vi "LVJSON Pop.vi"(8 "error in (no error)":errorcluster, 10 "Root Path ([]=Root)":string[](array[string]), 11 "Root Element in":T1) -> (0 "error out":errorcluster, 1 "Element out":T1, 2 "Exists?":bool, 3 "Root Element out":T1)   [LabVIEW 2018, in "labview_json.lvlib"]
uses:
  labview_json.lvlib
  Element Type.ctl
  Element.ctl
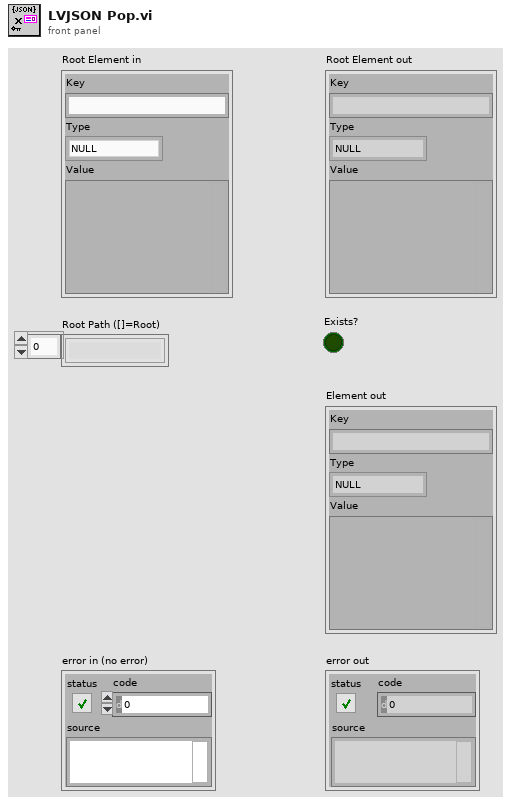
[diagram p1: front panel]
types:
  T1 = typedef "labview_json.lvlib/Element.ctl" = cluster{"Key":string, "Type":T2, "Value":variant}
  T2 = typedef "labview_json.lvlib/Element Type.ctl" = enum8{"NULL", "BOOL", "INT", "UINT", "FLOAT", "STRING", "ARRAY", "OBJECT", "SKIP"}
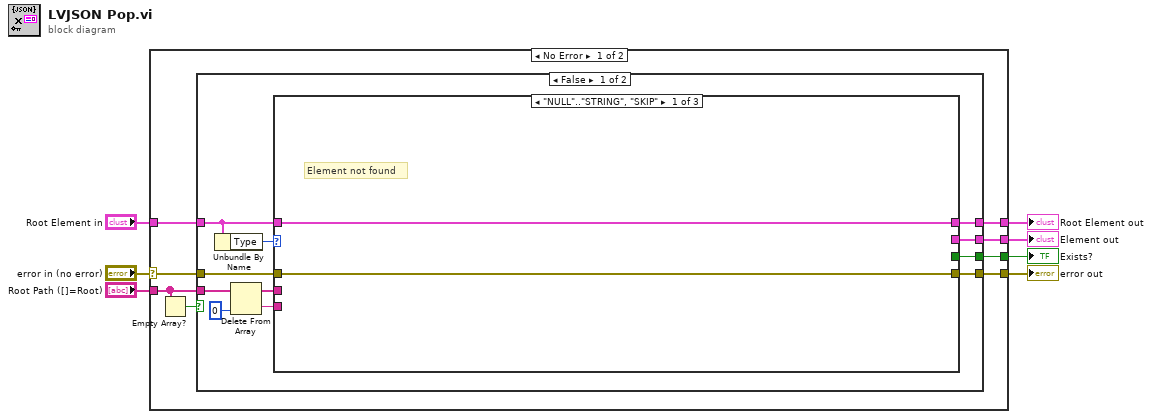
[diagram p0: block diagram]
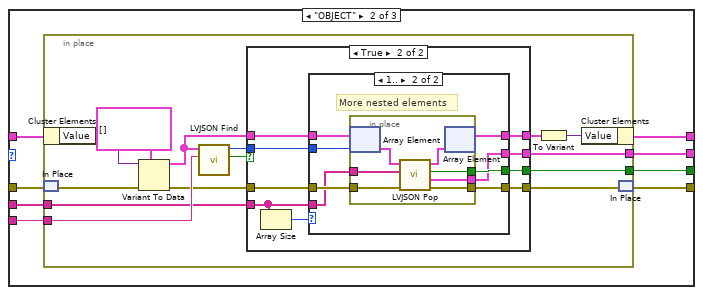
[diagram p2: hidden frame]
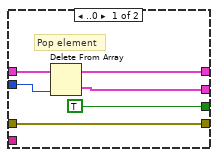
[diagram p4: hidden frame]
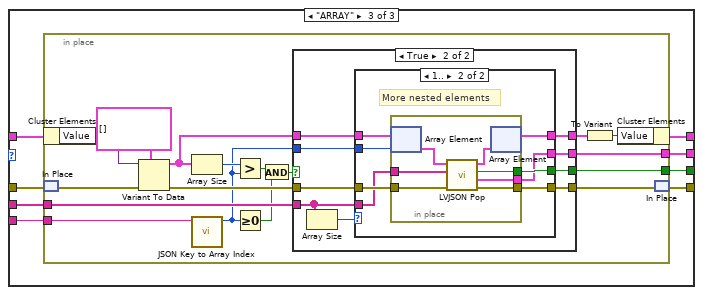
[diagram p5: hidden frame]
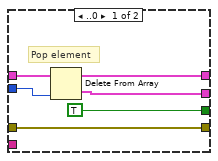
[diagram p7: hidden frame]
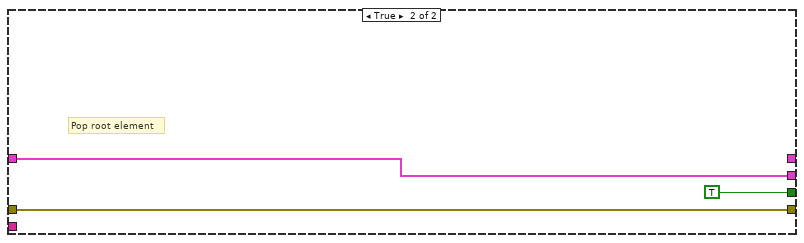
[diagram p8: hidden frame]
diagram:
  n1 = case shown="No Error" "error in (no error)" {
    selector: "error in (no error)" -> [w15 w144]
    tunnel: "Root Path ([]=Root)" -> [w9 _]
    tunnel: [w14 w144] -> w6
    tunnel: [w12 _] -> w5
    tunnel: [w13 _] -> w4
    tunnel: [w10 w143] -> w2
    tunnel: "Root Element in" -> [w11 w143]
    frame No Error {
      n2 = Empty Array?(array=w9) -> (empty?=w8:bool)
      n3 = case shown="False" w8 {
        tunnel: w15 -> [w26 w140]
        tunnel: [w25 w140] -> w14
        tunnel: [w24 TRUE ("Exists?")] -> w13
        tunnel: [w23 w142] -> w12
        tunnel: w11 -> [w22 w142]
        tunnel: w9 -> [w21 _]
        tunnel: [w20 _] -> w10
        frame False {
          n4 = Unbundle By Name(w22) -> ("Type"=w17:T2)
          n5 = Delete From Array(array=w21, index=0) -> (deleted portion=w16:string, array with subset deleted=w19:string[])  [unwired: 1 in]
          n6 = case shown="\"NULL\"..\"STRING\", \"SKIP\"" w17 {
            tunnel: w16 -> [_ w36 w90]
            tunnel: w26 -> [w28 w34 w88]
            tunnel: [w28 w33 w87] -> w25
            tunnel: [_ w29 w83] -> w23
            tunnel: w22 -> [w27 w35 w89]
            tunnel: [_ w30 w84] -> w24
            tunnel: w19 -> [_ w31 w85]
            tunnel: [w27 w32 w86] -> w20
            frame "NULL".."STRING", "SKIP" {
              # "Element not found"
            }
            frame "OBJECT" {
              n7 = in-place {
                in-place-border: w36 -> [w49]
                in-place-border: w31 -> [w40]
                in-place-border: [w38] -> w30
                in-place-border: [w37] -> w29
                n8 = in-place-cluster #1(w35) -> ("Value"=w45:variant)
                n9 = in-place-match #2(w34) -> (w44:errorcluster)
                n10 = Variant To Data(error in=w44, type=T1[] [] ("Values"), Variant=w45) -> (data=w47:T1[], error out=w48:errorcluster)
                n11 = call "LVJSON Find.vi"("Key"=w49, "Elements in"=w47) -> ("Found?"=w39:bool, "Index"=w46:i32)  [unwired: 8 in]
                n12 = case shown="True" w39 {
                  tunnel: w48 -> [w51 w61]
                  tunnel: w47 -> [w52 w60]
                  tunnel: w46 -> [_ w59]
                  tunnel: [w51 w58] -> w43
                  tunnel: [w52 w57] -> w42
                  tunnel: w40 -> [_ w56]
                  tunnel: [_ w53] -> w38
                  tunnel: [_ w54] -> w37
                  frame False {
                    # "Key does not exist"
                  }
                  frame True {
                    n13 = Array Size(array=w56) -> (size(s)=w55:i32)
                    n14 = case shown="1.." w55 {
                      tunnel: w61 -> [w62 w75]
                      tunnel: w60 -> [w67 w74]
                      tunnel: w59 -> [w66 w73]
                      tunnel: [w62 w72] -> w58
                      tunnel: [w65 w71] -> w57
                      tunnel: w56 -> [_ w70]
                      tunnel: [w64 w68] -> w54
                      tunnel: [TRUE w69] -> w53
                      frame ..0 {
                        # "Pop element"
                        n15 = Delete From Array(array=w67, index=w66) -> (deleted portion=w64:T1, array with subset deleted=w65:T1[])  [unwired: 1 in]
                      }
                      frame 1.. {
                        # "More nested elements"
                        n16 = in-place {
                          in-place-border: [w82] -> w72
                          in-place-border: w75 -> [w81]
                          in-place-border: w70 -> [w80]
                          in-place-border: [w77] -> w69
                          in-place-border: [w76] -> w68
                          n17 = in-place-array #3(w74, w73) -> (w79:T1)
                          n18 = call "LVJSON Pop.vi"("error in (no error)"=w81, "Root Path ([]=Root)"=w80, "Root Element in"=w79) -> ("error out"=w82:errorcluster, "Element out"=w76:T1, "Exists?"=w77:bool, "Root Element out"=w78:T1)  [unwired: 5 in]
                          n19 = in-place-array #3(w78) -> (w71:T1[])  [unwired: 1 out]
                        }
                      }
                    }
                  }
                }
                n20 = To Variant(anything=w42) -> (Variant=w41:variant)
                n21 = in-place-cluster #1("Value"=w41) -> (w32:T1)
                n22 = in-place-match #2(w43) -> (w33:errorcluster)
              }
            }
            frame "ARRAY" {
              n23 = in-place {
                in-place-border: w90 -> [w97]
                in-place-border: w85 -> [w100]
                in-place-border: [w99] -> w84
                in-place-border: [w98] -> w83
                n24 = in-place-cluster #4(w89) -> ("Value"=w105:variant)
                n25 = in-place-match #5(w88) -> (w104:errorcluster)
                n26 = Variant To Data(error in=w104, type=T1[] [] ("Values"), Variant=w105) -> (data=w95:T1[], error out=w106:errorcluster)
                n27 = Array Size(array=w95) -> (size(s)=w94:i32)
                n28 = call "JSON Key to Array Index.vi"("Key"=w97) -> ("Index"=w91:i32)  [unwired: 8 in, 2 out]
                n29 = Greater?(x=w94, y=w91) -> (0:w93:bool)
                n30 = Greater Or Equal To 0?(x=w91) -> (x >= 0?=w96:bool)
                n31 = And(x=w93, y=w96) -> (x .and. y?=w92:bool)
                n32 = case shown="True" w92 {
                  tunnel: w106 -> [w108 w118]
                  tunnel: w95 -> [w109 w117]
                  tunnel: w91 -> [_ w116]
                  tunnel: [w108 w115] -> w103
                  tunnel: [w109 w114] -> w102
                  tunnel: w100 -> [_ w113]
                  tunnel: [_ w110] -> w99
                  tunnel: [_ w111] -> w98
                  frame False {
                    # "Index does not exist"
                  }
                  frame True {
                    n33 = Array Size(array=w113) -> (size(s)=w112:i32)
                    n34 = case shown="1.." w112 {
                      tunnel: w118 -> [w119 w132]
                      tunnel: w117 -> [w124 w131]
                      tunnel: w116 -> [w123 w130]
                      tunnel: [w119 w129] -> w115
                      tunnel: [w122 w128] -> w114
                      tunnel: w113 -> [_ w127]
                      tunnel: [w121 w125] -> w111
                      tunnel: [TRUE w126] -> w110
                      frame ..0 {
                        # "Pop element"
                        n35 = Delete From Array(array=w124, index=w123) -> (deleted portion=w121:T1, array with subset deleted=w122:T1[])  [unwired: 1 in]
                      }
                      frame 1.. {
                        # "More nested elements"
                        n36 = in-place {
                          in-place-border: [w139] -> w129
                          in-place-border: w132 -> [w138]
                          in-place-border: w127 -> [w137]
                          in-place-border: [w134] -> w126
                          in-place-border: [w133] -> w125
                          n37 = in-place-array #6(w131, w130) -> (w136:T1)
                          n38 = call "LVJSON Pop.vi"("error in (no error)"=w138, "Root Path ([]=Root)"=w137, "Root Element in"=w136) -> ("error out"=w139:errorcluster, "Element out"=w133:T1, "Exists?"=w134:bool, "Root Element out"=w135:T1)  [unwired: 5 in]
                          n39 = in-place-array #6(w135) -> (w128:T1[])  [unwired: 1 out]
                        }
                      }
                    }
                  }
                }
                n40 = To Variant(anything=w102) -> (Variant=w101:variant)
                n41 = in-place-cluster #4("Value"=w101) -> (w86:T1)
                n42 = in-place-match #5(w103) -> (w87:errorcluster)
              }
            }
          }
        }
        frame True {
          # "Pop root element"
        }
      }
    }
    frame Error {
    }
  }
  "error out" <- w6
  "Exists?" <- w4
  "Element out" <- w5
  "Root Element out" <- w2
